vi "RT Main.vi"   [LabVIEW 2013]
doc: "本模板用于队列消息处理器设计模式。\n\n事件处理循环负责按用户界面操作生成对应的消息。\n\n消息处理循环负责对事件处理循环或其他消息生成的消息进行处理。消息内容为字符串值，因此很容易将新消息添加至“消息处理”循环的“消息分支”条件结构。每个消息簇还可选择性地为消息数据提供一个变体，变体数据可以转换为消息数据所需要的任意类型。"
uses:
  Globals/Global - All RT Loop Stop.vi
  Globals/Global - Configuration Options.vi
  support/Message Queue/Message Queue.lvlib
  <vilib>/nisyscfg/nisyscfg.lvlib
types:
  T1 = typedef "Acquisition and Logging Configuration.ctl" = cluster{"Samples per Read":i32, "Number of Reads to Save":i32, "Number of Channels":i32, "Channel Scale Array":fxp<+,24,12>[], "Channel Names":string[], "Trigger - RMS Value":dbl, "Trigger - Channel":i32, "Trigger - Time (Minute)":i32, "TDMS Properties":T2[], "Data File Name":string, "Date Rate":T3}
  T2 = typedef "TDMS Properties.ctl" = cluster{"Name":string, "Value":string}
  T3 = typedef "nicrio_cRIO-9234_DataRatesRing2.ctl" = u16
  T4 = typedef "Message Queue.lvlib/All Real-Time Message Queues.ctl" = cluster{"Message Handler":refnum<queue>, "Acquisition and Logging":refnum<queue>}
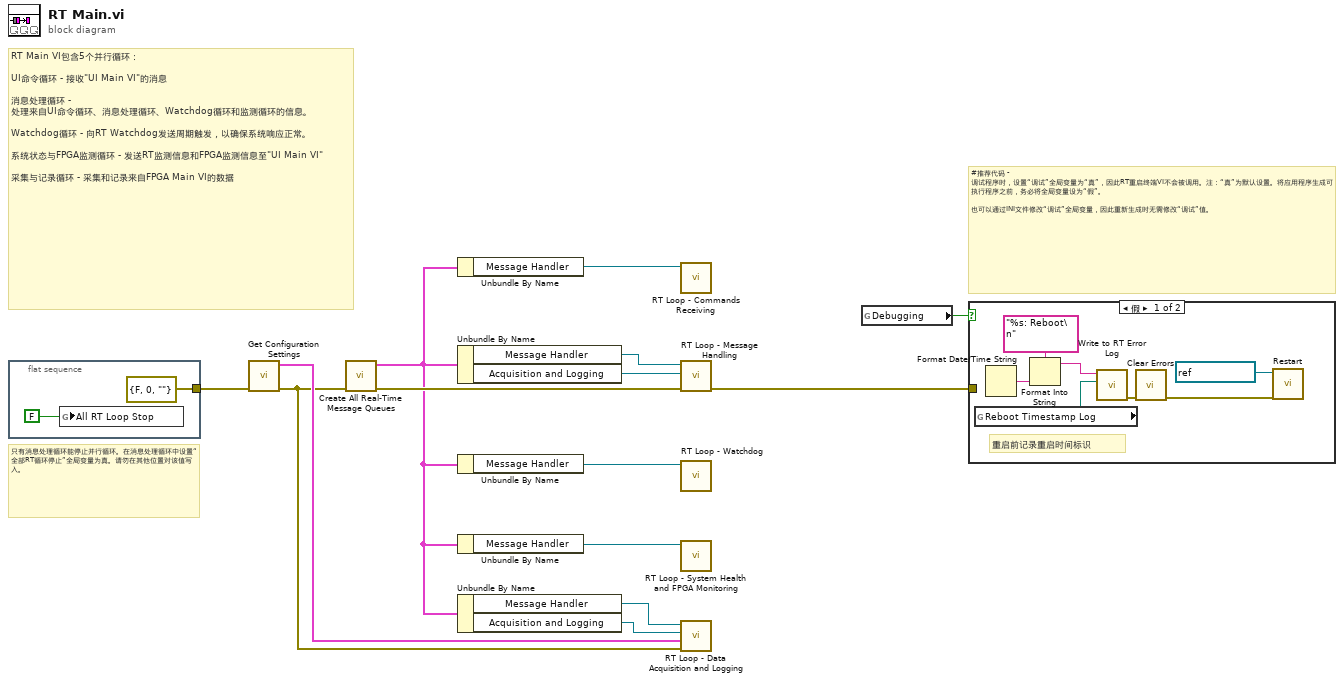
[diagram p0: block diagram]
diagram:
  # "#推荐代码 - 调试程序时，设置“调试”全局变量为“真”，因此RT重启终端VI不会被调用。注：“真”为默认设置。将应用程序生成可执行程序之前，务必将全局变量设为“假”。\n\n也可以通过INI文件修改“调试”全局变量，因此重新生成时无需修改“调试”值。"
  # "RT Main VI包含5个并行循环：\n\nUI命令循环 - 接收\"UI Main VI\"的消息\n\n消息处理循环 - 处理来自UI命令循环、消息处理循环、Watchdog循环和监测循环的信息。\n\nWatchdog循环 - 向RT Watchdog发送周期触发，以确保系统响应正常。\n\n系统状态与FPGA监测循环 - 发送RT监测信息和FPGA监测信息至\"UI Main VI\"\n\n采集与记录循环 - 采集和记录来自FPGA Main VI的数据"
  # "只有消息处理循环能停止并行循环。在消息处理循环中设置“全部RT循环停止”全局变量为真。请勿在其他位置对该值写入。"
  n1 = flat-sequence {
    tunnel: [errorcluster {"status"=FALSE, "code"=0, "source"=""} ("error constant")] -> w14
    frame #0 {
      n2 = global write "Global - All RT Loop Stop.vi" "All RT Loop Stop"(FALSE) -> ()
    }
  }
  n3 = call "Get Configuration Settings.vi"("error in (no error)"=w14) -> ("error out"=w2:errorcluster, "Acquisition and Logging Configuration"=w11:T1)  [unwired: 9 in]
  n4 = call "Create All Real-Time Message Queues.vi"("error in (no error)"=w2) -> ("error out"=w10:errorcluster, "Message Queues out"=w9:T4)  [unwired: 9 in]
  n5 = Unbundle By Name(w9) -> ("Message Handler"=w5:refnum<queue>)
  n6 = Unbundle By Name(w9) -> ("Message Handler"=w1:refnum<queue>, "Acquisition and Logging"=w3:refnum<queue>)
  n7 = Unbundle By Name(w9) -> ("Message Handler"=w8:refnum<queue>)
  n8 = Unbundle By Name(w9) -> ("Message Handler"=w7:refnum<queue>)
  n9 = Unbundle By Name(w9) -> ("Message Handler"=w6:refnum<queue>, "Acquisition and Logging"=w4:refnum<queue>)
  n10 = call "RT Loop - Commands Receiving.vi"("Message Queue"=w5) -> ()  [unwired: 11 in]
  n11 = call "RT Loop - Message Handling.vi"("error in (no error)"=w10, "A&L Message Queue"=w3, "Control Message Queue"=w1) -> ("error out"=w13:errorcluster)  [unwired: 8 in]
  n12 = call "RT Loop - Watchdog.vi"("Message Queue"=w8) -> ()  [unwired: 11 in]
  n13 = call "RT Loop - System Health and FPGA Monitoring.vi"("Message Queue"=w7) -> ()  [unwired: 11 in]
  n14 = call "RT Loop - Data Acquisition and Logging.vi"("error in (no error)"=w2, "Acquisition and Logging Configuration"=w11, "Acquisition and Logging Queue"=w4, "Message Queue"=w6) -> ()  [unwired: 7 in, 1 out]
  n15 = global read "Global - Configuration Options.vi" "Debugging"() -> (w12:bool)
  n16 = case shown="假" w12 {
    tunnel: w13 -> [_ _]
    frame False {
      # "重启前记录重启时间标识"
      n17 = global read "Global - Configuration Options.vi" "Reboot Timestamp Log"() -> (w19:path)
      n18 = Format Date/Time String() -> (date/time string=w21:string)  [unwired: 3 in]
      n19 = Format Into String(format string="%s: Reboot\n", w21) -> (resulting string=w20:string)  [unwired: 2 in, 1 out]
      n20 = call "Write to RT Error Log.vi"("Error Log Path"=w19, "Log Entry"=w20) -> ("error out"=w23:errorcluster)  [unwired: 9 in]
      n21 = call <vilib>:"Clear Errors.vi"("error in (no error)"=w23) -> ("error out"=w18:errorcluster)  [unwired: 6 in]
      n22 = call <vilib>:"Restart.vi"("error in (no error)"=w18, "session in"=refnum<k21> "localhost") -> ()  [unwired: 7 in, 3 out]
    }
    frame True {
    }
  }
